vi "save.vi"(0 "M1M3Settings in":refnum<class "TCSettings.lvclass">, 11 "error in (no error)":errorcluster) -> (4 "M1M3Settings out":refnum<class "TCSettings.lvclass">, 10 "Canceled":bool, 15 "error out":errorcluster)   [LabVIEW 2016, in "Settings.lvlib" / "TCSettings.lvclass"]
uses:
  TCSettings.lvclass
  home/harini/tcs/ct_cmpuserevents/ComponentTemplateCore/Settings/Settings/Setting.lvclass
  Settings/Setting.lvclass/Setting.ctl
  Settings/Setting.lvclass
panel:
  in  "UseNewSetting":bool
  in  "UseAvailableSetting":bool=TRUE
  in  "New Setting":string
  in  "Cancel":bool
  in  "Save":bool
  in  "Available Settings":i32(listbox)
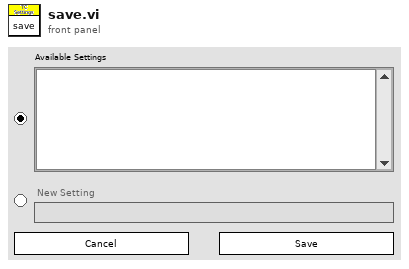
[diagram p1: front panel]
types:
  T1 = enum8{"Enabled", "Disabled", "Disabled and Grayed Out"}
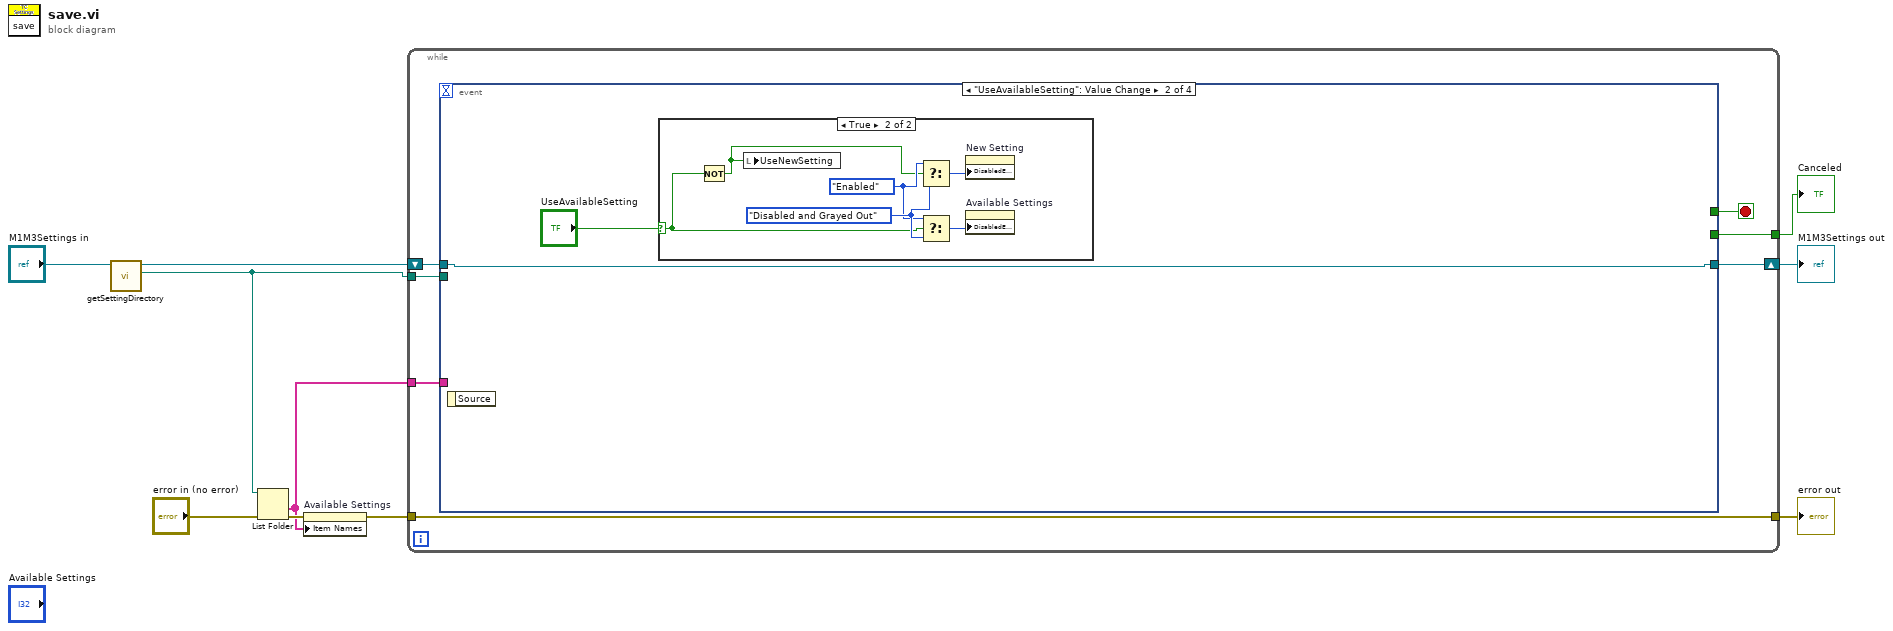
[diagram p0: block diagram]
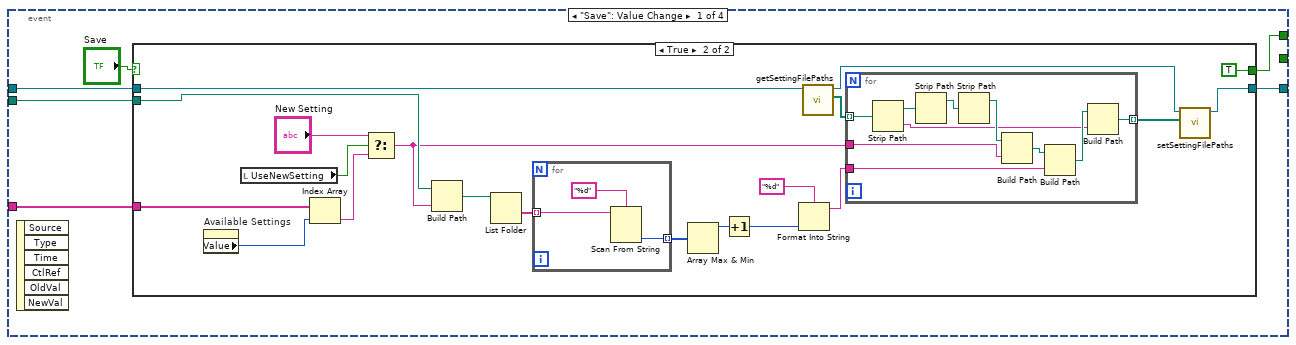
[diagram p2: hidden frame]
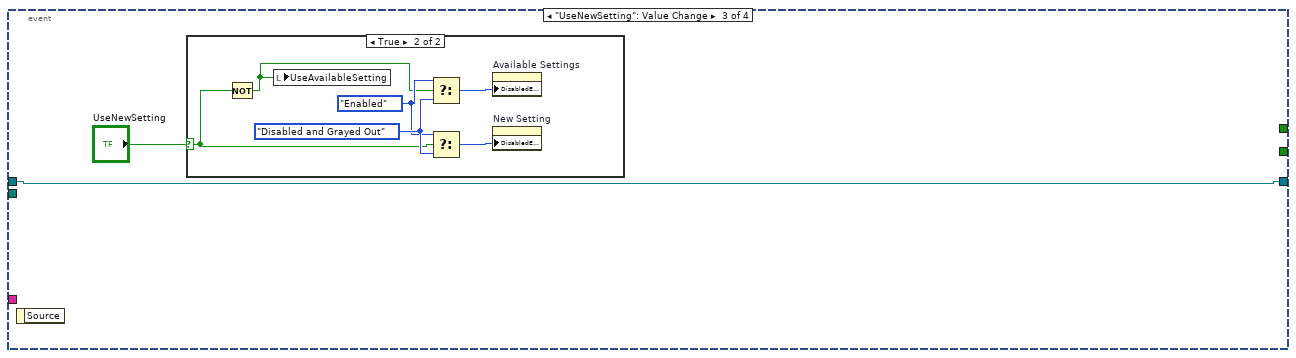
[diagram p5: hidden frame]
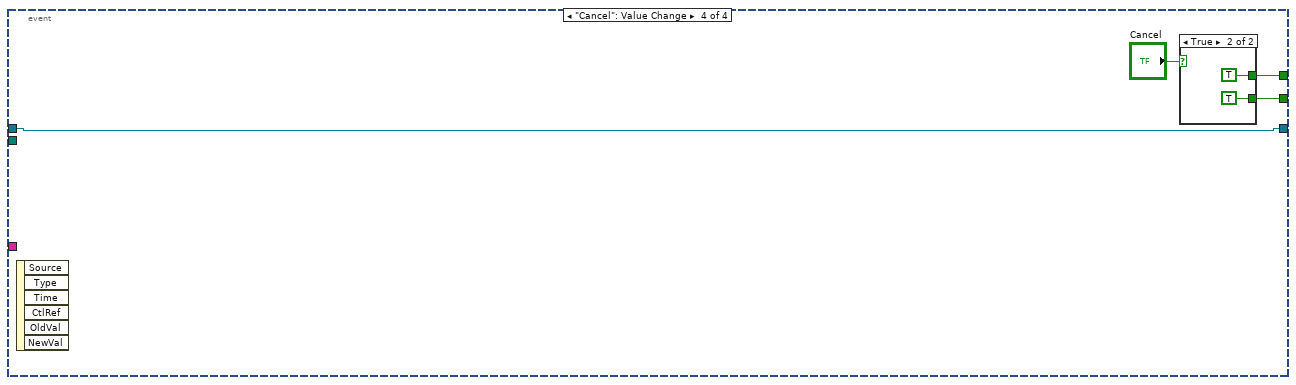
[diagram p7: hidden frame]
diagram:
  n1 = call "getSettingDirectory.vi"("BaseSetting in"="M1M3Settings in") -> ("SettingDirectory"=w1:path, "BaseSetting out"=w3:refnum<class "TCSettings.lvclass">)  [unwired: 9 in]
  n2 = List Folder(path=w1, error in="error in (no error)") -> (folder names=w5:string[], error out=w6:errorcluster)  [unwired: 2 in, 2 out]
  n3 = property on="Available Settings" class="LstBox (strict)"(error in=w6, "Item Names"=w5) -> (error out=w8:errorcluster)  [unwired: 1 in, 1 out]
  n4 = while {
    tunnel: [w16] -> w4
    tunnel: [w15] -> w9
    tunnel: w8 -> [w15]
    tunnel: w5 -> [w14]
    tunnel: w1 -> [w13]
    shift-right: [w12] -> w2
    shift-left: w3 -> [w11]
    stop <- w17 stop-if-true
    n5 = event shown="[1] \"UseAvailableSetting\": Value Change" {
      selector: _ -> [_ _ _ _]
      dyn-events: _ -> [_ _ _ _]
      timeout: _ -> [_ _ _ _]
      tunnel: [w22 _ _ w76] -> w17
      tunnel: [_ _ _ w75] -> w16
      tunnel: w14 -> [w21 _ _ _]
      tunnel: w13 -> [w20 _ _ _]
      tunnel: [w19 w59 w67 w74] -> w12
      tunnel: w11 -> [w18 w59 w67 w74]
      event "Save": Value Change {
        n6 = event-data() -> ()  [unwired: 1 in, 6 out]
        n7 = case shown="True" "Save" {
          tunnel: [_ TRUE] -> w22
          tunnel: w21 -> [_ w40]
          tunnel: w20 -> [_ w38]
          tunnel: [w24 w34] -> w19
          tunnel: w18 -> [w24 w33]
          frame False {
          }
          frame True {
            n8 = property on="Available Settings" class="LstBox (strict)"() -> ("Value"=w41:i32)  [unwired: 2 in, 2 out]
            n9 = local read "UseNewSetting"() -> (w42:bool)
            n10 = Index Array(array=w40, index=w41) -> (element=w39:string)
            n11 = Select(t="New Setting", s=w42, f=w39) -> (s? t:f=w37:string)
            n12 = Build Path(base path=w38, name or relative path=w37) -> (appended path=w30:path)
            n13 = List Folder(path=w30) -> (folder names=w29:string[])  [unwired: 3 in, 3 out]
            n14 = for {
              tunnel: w29 -> [w47] mode=indexing
              tunnel: [w45] -> w28 mode=indexing
              n15 = Scan From String(format string="%d", input string=w47) -> (output 1=w45:i32)  [unwired: 3 in, 3 out]
            }
            n16 = Array Max & Min(array=w28) -> (max value=w27:i32)  [unwired: 3 out]
            n17 = Increment(x=w27) -> (x+1=w25:i32)
            n18 = Format Into String(format string="%d", w25) -> (resulting string=w36:string)  [unwired: 2 in, 1 out]
            n19 = call "getSettingFilePaths.vi"("Setting in"=w33) -> ("SettingFilePaths"=w32:path[], "Setting out"=w31:refnum<class "TCSettings.lvclass">)  [unwired: 9 in]
            n20 = for {
              tunnel: w32 -> [w57] mode=indexing
              tunnel: w37 -> [w53]
              tunnel: w36 -> [w51]
              tunnel: [w48] -> w35 mode=indexing
              n21 = Strip Path(path=w57) -> (stripped path=w56:path, name=w49:string)
              n22 = Strip Path(path=w56) -> (stripped path=w55:path)  [unwired: 1 out]
              n23 = Strip Path(path=w55) -> (stripped path=w54:path)  [unwired: 1 out]
              n24 = Build Path(base path=w54, name or relative path=w53) -> (appended path=w52:path)
              n25 = Build Path(base path=w52, name or relative path=w51) -> (appended path=w50:path)
              n26 = Build Path(base path=w50, name or relative path=w49) -> (appended path=w48:path)
            }
            n27 = call "setSettingFilePaths.vi"("SettingFilePaths"=w35, "Setting in"=w31) -> ("Setting out"=w34:refnum<class "TCSettings.lvclass">)  [unwired: 9 in]
          }
        }
      }
      event "UseAvailableSetting": Value Change {
        n28 = event-data() -> ()  [unwired: 1 in, 1 out]
        n29 = case shown="True" "UseAvailableSetting" {
          selector: "UseAvailableSetting" -> [_ w60]
          frame False {
          }
          frame True {
            w64 = T1."Disabled and Grayed Out" ("f")
            w63 = T1."Enabled" ("Disabled")
            n30 = Not(x=w60) -> (.not. x?=w62:bool)
            n31 = local write "UseNewSetting"(w62) -> ()
            n32 = Select(t=w63, s=w62, f=w64) -> (s? t:f=w61:T1)
            n33 = Select(t=w63, s=w60, f=w64) -> (s? t:f=w65:T1)
            n34 = property on="New Setting" class="Str"("DisabledEnum"=w61) -> ()  [unwired: 2 in, 2 out]
            n35 = property on="Available Settings" class="LstBox (strict)"("DisabledEnum"=w65) -> ()  [unwired: 2 in, 2 out]
          }
        }
      }
      event "UseNewSetting": Value Change {
        n36 = event-data() -> ()  [unwired: 1 in, 1 out]
        n37 = case shown="True" "UseNewSetting" {
          selector: "UseNewSetting" -> [_ w68]
          frame False {
          }
          frame True {
            w72 = T1."Disabled and Grayed Out" ("f")
            w71 = T1."Enabled" ("Disabled")
            n38 = Not(x=w68) -> (.not. x?=w70:bool)
            n39 = local write "UseAvailableSetting"(w70) -> ()
            n40 = Select(t=w71, s=w70, f=w72) -> (s? t:f=w69:T1)
            n41 = Select(t=w71, s=w68, f=w72) -> (s? t:f=w73:T1)
            n42 = property on="Available Settings" class="LstBox (strict)"("DisabledEnum"=w69) -> ()  [unwired: 2 in, 2 out]
            n43 = property on="New Setting" class="Str"("DisabledEnum"=w73) -> ()  [unwired: 2 in, 2 out]
          }
        }
      }
      event "Cancel": Value Change {
        n44 = event-data() -> ()  [unwired: 1 in, 6 out]
        n45 = case shown="True" "Cancel" {
          tunnel: [_ TRUE] -> w76
          tunnel: [_ TRUE] -> w75
          frame False {
          }
          frame True {
          }
        }
      }
    }
  }
  "error out" <- w9
  "M1M3Settings out" <- w2
  "Canceled" <- w4
